vi "AOsource.vi"(9 "last value":dbl[](array[numeric]) format="%.2f", 10 "waveforms in":T2 format="%.2f", 11 "AO":T1={"n"=1, "on/off"=[]} {"n" min=1}) -> (3 "waveforms out":sgl[][](array[numeric]) format="%.2f")   [LabVIEW 2010]
uses:
  wavecluster.ctl
  AO n wave.ctl
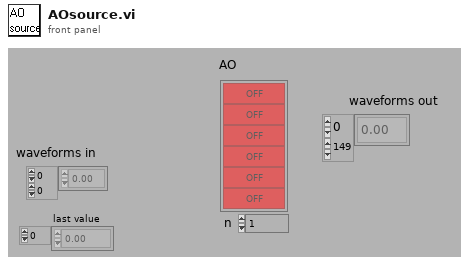
[diagram p1: front panel]
types:
  T1 = typedef "AO n wave.ctl" = cluster{"n":i32, "on/off":bool[]}
  T2 = typedef "wavecluster.ctl" = sgl[][]
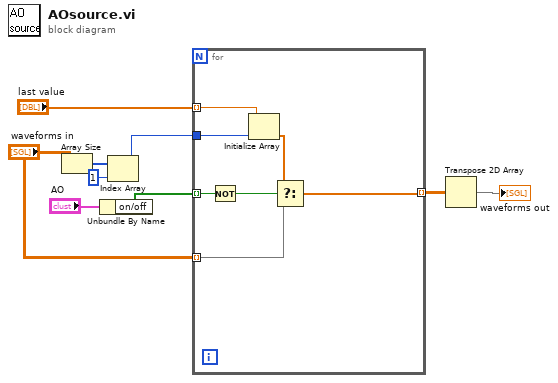
[diagram p0: block diagram]
diagram:
  n1 = Array Size(array="waveforms in") -> (size(s)=w7:i32[])
  n2 = Unbundle By Name("AO") -> ("on/off"=w3:bool[])
  n3 = Index Array(array=w7, index=1) -> (element=w5:i32)
  n4 = for {
    tunnel: "last value" -> [w16] mode=indexing
    tunnel: w5 -> [w15]
    tunnel: "waveforms in" -> [w14] mode=indexing
    tunnel: w3 -> [w12] mode=indexing
    tunnel: [w11] -> w2 mode=indexing
    n5 = Not(x=w12) -> (.not. x?=w10:bool)
    n6 = Initialize Array(w16, w15) -> (w13:dbl[])
    n7 = Select(t=w13, s=w10, f=w14) -> (s? t:f=w11:dbl[])
  }
  n8 = Transpose 2D Array(2D array=w2) -> (transposed array=→"waveforms out":dbl[][])
